vi "ClearFP.vi"(8 "error in":errorcluster, 11 "reference":refnum<vi>) -> (0 "error out":errorcluster, 3 "reference out":refnum<vi>)   [LabVIEW 2013, in "data interface script.lvlib"]
uses:
  data interface script.lvlib
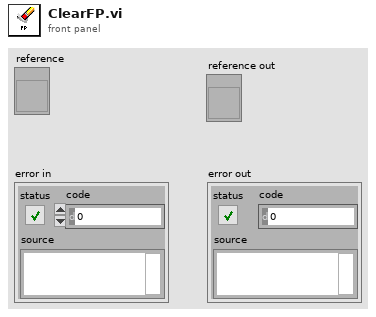
[diagram p1: front panel]
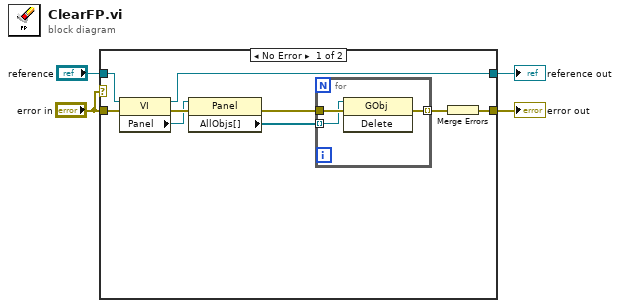
[diagram p0: block diagram]
diagram:
  n1 = case shown="No Error" "error in" {
    tunnel: "reference" -> [w12 w18]
    tunnel: "error in" -> [w11 w17]
    tunnel: [w10 w18] -> w3
    tunnel: [w9 w17] -> w2
    frame No Error {
      n2 = property class="VI"(reference=w12, error in=w11) -> (reference out=w10:refnum<vi>, error out=w8:errorcluster, "Panel"=w7:refnum<vi>)
      n3 = property class="Panel"(reference=w7, error in=w8) -> (error out=w6:errorcluster, "AllObjs[]"=w5:refnum<vi>[])  [unwired: 1 out]
      n4 = for {
        tunnel: w6 -> [w16]
        tunnel: w5 -> [w15] mode=indexing
        tunnel: [w14] -> w13 mode=indexing
        n5 = invoke class="GObj" method="Delete"(reference=w15, error in=w16) -> (error out=w14:errorcluster)  [unwired: 1 in, 2 out]
      }
      n6 = Merge Errors(w13) -> (w9:errorcluster)
    }
    frame Error {
    }
  }
  "reference out" <- w3
  "error out" <- w2
